vi "ref_forcecontrol_pitchmotor_pid_sensor.vi"() -> ()   [LabVIEW 2014]
uses:
  <vilib>/rvi/FXPMathLib/FxpSinAndCos/XNode/nifxpmath_SinAndCos.xnode
  <vilib>/eio/EIONode/EIONode.xnode
  <vilib>/rvi/FXPMathLib/FxpMul/XNode/nifxpmath_Multiplier.xnode
  <vilib>/rvi/FXPMathLib/FxpSinAndCos/simVIs/DllFxpSinAndCosTemp_sub.vi
  <vilib>/rvi/FXPMathLib/FxpSinAndCos/subVIs/nifxpmath_SinAndCos_SimConfig.ctl
  <vilib>/rvi/eio/common/nirviEmuTemplateMethod_errors.vi
  <vilib>/rvi/FXPMathLib/sim/FxpSim.dll
  <vilib>/rvi/DataTransferAndStorage/Container/XNode/niFpgaContainer.xnode
  <vilib>/rvi/FXPMathLib/FxpSub/XNode/nifxpmath_Sub.xnode
  <vilib>/rvi/FXPMathLib/FxpAdd/XNode/nifxpmath_Add.xnode
  <vilib>/rvi/Analysis/measure/butterworth/XNode/niFpgaButterworthFilter.xnode
  <vilib>/eio/EIOPropertyNode/EIOPropertyNode.xnode
  <vilib>/rvi/eio/common/nirviEmuTemplatePropertyGet_errors.vi
  <vilib>/rvi/eio/common/nirviEmuTemplatePropertyGet_noerrors.vi
  <vilib>/rvi/eio/common/nirviEmuTemplatePropertySet_errors.vi
  <vilib>/rvi/eio/common/nirviEmuTemplatePropertySet_noerrors.vi
  <vilib>/rvi/interface/RandomDataEmulation/nirviRandomDataFpgaReadWriteTemplate.vi
  <vilib>/LabVIEW Targets/FPGA/cRIO/shared/nicrio_ModuleControls/nicrio_cRIO-9237_DataRatesRing.ctl
  <vilib>/LabVIEW Targets/FPGA/cRIO/shared/nicrio_ModuleControls/nicrio_cRIO-9237_ExcitationVoltageRing.ctl
panel:
  in  "Unstrained Measurements_p":fxp<+/-,22,1>
  in  "LRCF_p":fxp<+,22,1>
  in  "Unstrained Measurements_y":fxp<+/-,22,1>
  in  "LRCF_y":fxp<+,22,1>
  in  "Fey_reset":bool
  out "Gauge_Fey":fxp<+/-,24,-4>
  in  "Gauge_stop":bool
  in  "Fep_reset":bool
  out "Gauge_Fep":fxp<+/-,24,-4>
  in  "Excitation Voltage":T1 items=["2.5 Volts", "3.3 Volts", "5.0 Volts", "10.0 Volts", "External Excitation"]
  in  "Data Rate":T2=1 items=["50.000 kS/s (NI 9237)"=1, "25.000 kS/s (NI 9237)"=2, "16.667 kS/s (NI 9237)"=3, "12.500 kS/s (NI 9237)"=4, "10.000 kS/s (NI 9237)"=5, "8.333 kS/s (NI 9237)"=6, "7.143 kS/s (NI 9237)"=7, "6.250 kS/s (NI 9237)"=8, "5.556 kS/s (NI 9237)"=9, "5.000 kS/s (NI 9237)"=10, "4.545 kS/s (NI 9237)"=11, "4.167 kS/s (NI 9237)"=12, "3.846 kS/s (NI 9237)"=13, "3.571 kS/s (NI 9237)"=14, "3.333 kS/s (NI 9237)"=15, "3.125 kS/s (NI 9237)"=16, "2.941 kS/s (NI 9237)"=17, "2.778 kS/s (NI 9237)"=18, "2.632 kS/s (NI 9237)"=19, "2.500 kS/s (NI 9237)"=20, "2.381 kS/s (NI 9237)"=21, "2.273 kS/s (NI 9237)"=22, "2.174 kS/s (NI 9237)"=23, "2.083 kS/s (NI 9237)"=24, "2.000 kS/s (NI 9237)"=25, "1.923 kS/s (NI 9237)"=26, "1.852 kS/s (NI 9237)"=27, "1.786 kS/s (NI 9237)"=28, "1.724 kS/s (NI 9237)"=29, "1.667 kS/s (NI 9237)"=30, "1.613 kS/s (NI 9237)"=31]
  in  "Step_fp_start":bool
  in  "Count(mSec)":u32
  in  "Fpr_step":fxp<+/-,20,10>
  in  "Fpr_numofstep":i32
  in  "Fpr_ini":fxp<+/-,20,10>
  in  "coe_ini":bool
  in  "D_comp/tune_p":bool
  in  "kp t":fxp<+,15,8>
  in  "kp c":fxp<+,15,8>
  in  "Kpp gain":fxp<+,10,4>=0.40625
  in  "Kpp slope gain":fxp<+,20,1>=0.40625
  in  "Kdp 2":fxp<+,26,2>
  in  "Kip 2":fxp<+,27,10>
  in  "I_comp/tune_p":bool
  out "Kpp":fxp<+,12,6>
  out "Kdp":fxp<+,26,2> format="%.25g"
  out "Kip":fxp<+,27,10> format="%.21g"
  in  "tolerance_p":fxp<+,12,2>=1.0
  out "fpr":fxp<+/-,20,10>
  in  "viscous_cons_p":fxp<+/-,20,10>
  in  "fcp":fxp<+/-,15,6>
  in  "fvp":fxp<+,20,12>
  in  "fv_coeff. p":fxp<+,13,1>
  in  "Dp_d_tol":fxp<+,20,12>
  in  "fstp":fxp<+/-,15,6>
  out "Friction comp_p":fxp<+/-,20,10>
  out "Fp_PID":fxp<+/-,20,10>
  out "fp_tilde":fxp<+/-,21,11>
  out "fpt_d":fxp<+/-,25,15>
  out "xp_d":fxp<+/-,25,15>
  out "fpt_i":fxp<+/-,25,11>
  out "Dp_d":fxp<+/-,25,15>
  out "vd_p_F":fxp<+/-,20,5>
  out "vq_p_F":fxp<+/-,20,5> format="%.57g"
  in  "Stop motor_p":bool
  out "va_p":fxp<+/-,20,5> format="%.21g"
  out "vb_p":fxp<+/-,20,5> format="%.21g"
  out "omega_p":fxp<+/-,20,9>
  in  "Encoder Reset_p":bool
  out "Encoder Position_p":i32
  out "rad(NrTheta)_p":fxp<+/-,33,18> format="%.21g"
  out "Dp(mm)":fxp<+/-,22,7>
  out "x_p":fxp<+/-,30,6> format="%.40g"
  in  "Linear Sensor Reset":bool
  in  "kp":fxp<+,15,8>
  out "fp":fxp<+/-,20,10>
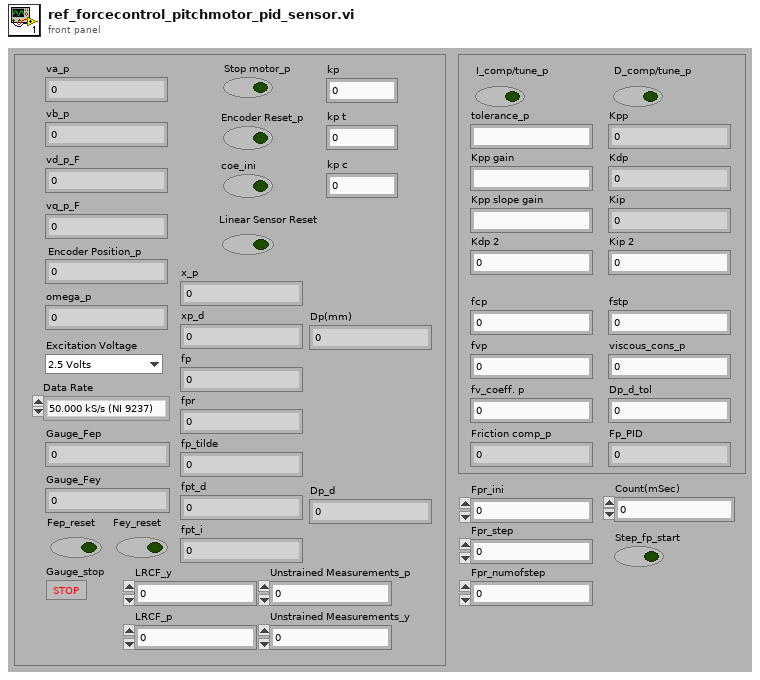
[diagram p1: front panel]
types:
  T1 = typedef "nicrio_cRIO-9237_ExcitationVoltageRing.ctl" = u8
  T2 = typedef "nicrio_cRIO-9237_DataRatesRing.ctl" = u8
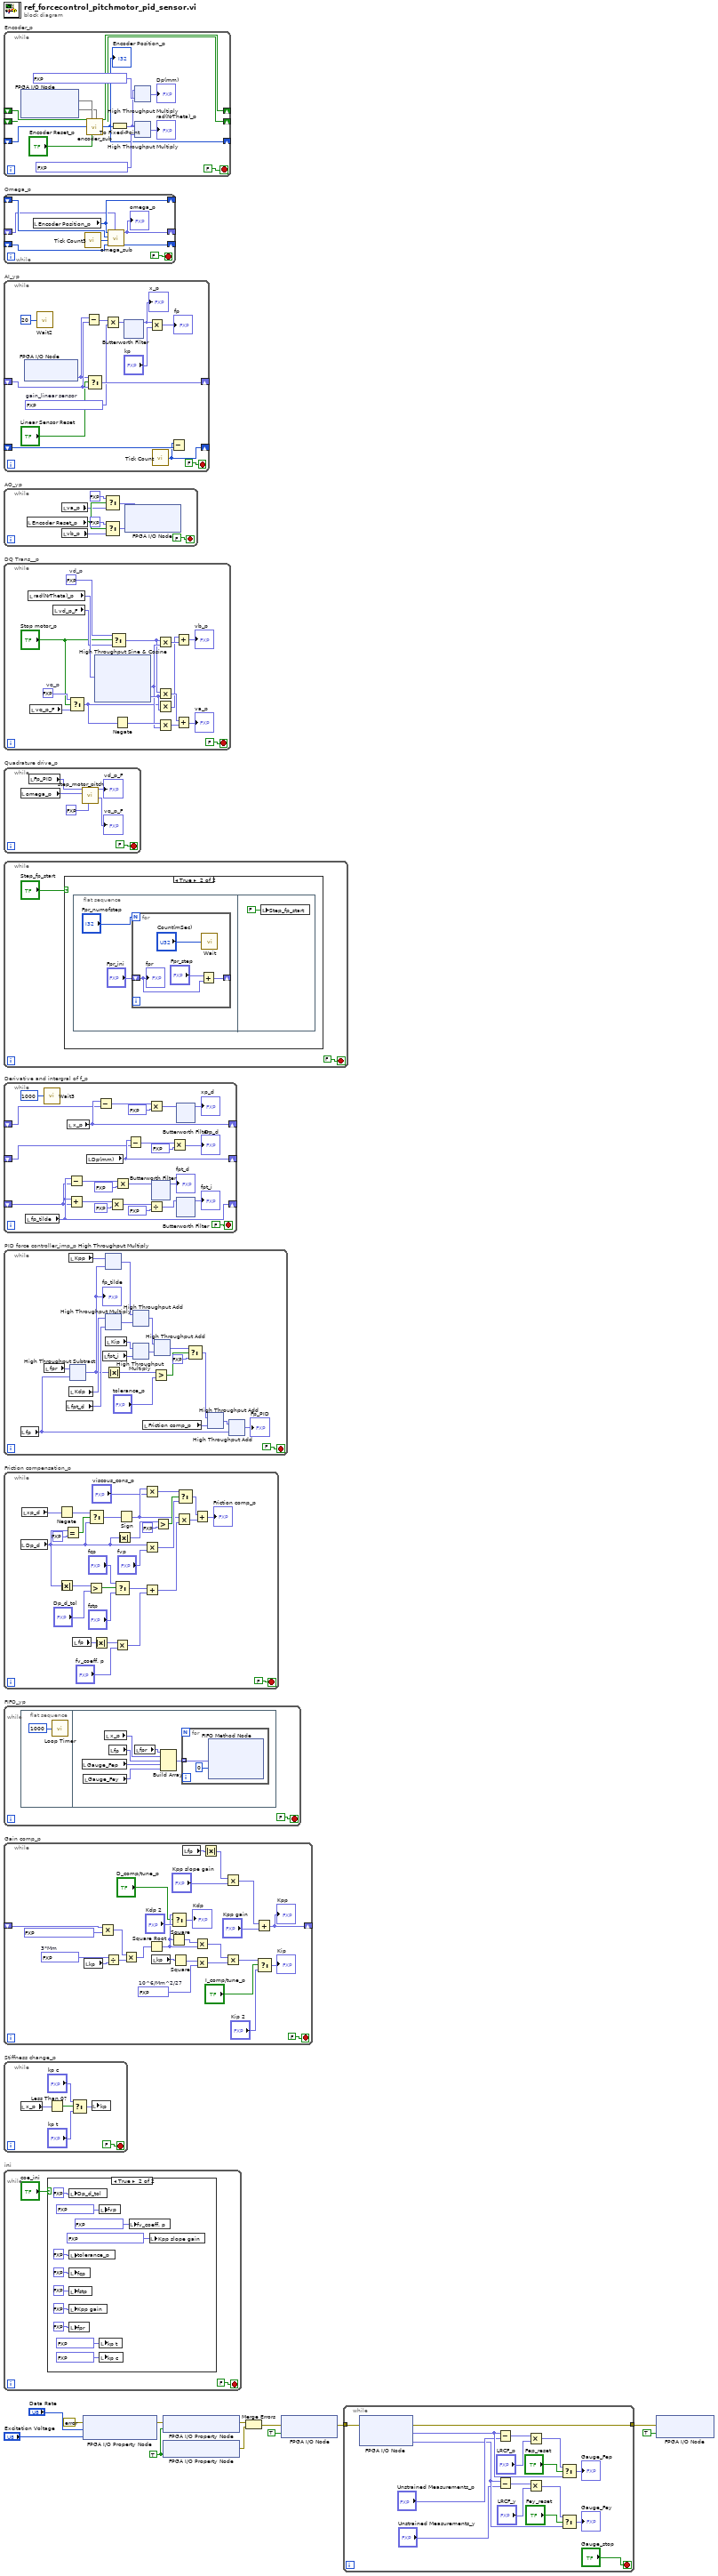
[diagram p0: block diagram]
diagram:
  w6 = TRUE ("Half-Bridge Enable")
  n1 = while "Encoder_p" {
    shift-right: [w26] -> _
    shift-left: _ -> [w24]
    shift-right: [w25] -> _
    shift-left: _ -> [w23]
    shift-right: [w13] -> _
    shift-left: _ -> [w19]
    stop <- FALSE stop-if-true
    n2 = xnode "FPGA I/O Node"() -> ("Mod3/DIO0"=w22, "Mod3/DIO1"=w21)  [unwired: 2 in, 2 out]
    n3 = call "encoder_sub.vi"("A_pre"=w24, "B_pre"=w23, "Encoder Position_pre"=w19, "A input"=w22, "Encoder Position Reset"="Encoder Reset_p", "B input"=w21) -> ("A"=w26:bool, "B"=w25:bool, "Encoder Position (Counts)"=w13:i32)  [unwired: 19 in]
    "Encoder Position_p" <- w13
    n4 = To Fixed-Point(number=w13) -> (fixed-point=w16:fxp<+/-,18,18>)  [unwired: 1 in]
    n5 = xnode ("High Throughput Multiply")("x"=w16, "y"=fxp<+/-,15,-9> -0.0006049871444702148) -> ("x*y"=→"Dp(mm)":fxp<+/-,21,6>)
    n6 = xnode ("High Throughput Multiply")("x"=w16, "y"=fxp<+,24,0> 0.02499997615814209) -> ("x*y"=→"rad(NrTheta)_p":fxp<+/-,33,18>)
  }
  n7 = while "Omega_p" {
    shift-right: [w35] -> _
    shift-left: _ -> [w34]
    shift-right: [w33] -> _
    shift-left: _ -> [w32]
    shift-right: [w30] -> _
    shift-left: _ -> [w31]
    stop <- FALSE stop-if-true
    n8 = local read "Encoder Position_p"() -> (w35:i32)
    n9 = call "Tick Count3"() -> ("Tick Count(Ticks)"=w28:u32)
    n10 = call "omega_sub.vi"("omega_pre"=w31, "ticks_m_pre"=w32, "ticks"=w28, "count_pre"=w34, "count"=w35) -> ("ticks_m"=w33:u32, "omega"=w30:fxp<+/-,20,9>)  [unwired: 4 in, 1 out]
    "omega_p" <- w30
  }
  n11 = while "AI_yp" {
    shift-right: [w48] -> _
    shift-left: _ -> [w49]
    shift-right: [w45] -> _
    shift-left: _ -> [w46]
    stop <- FALSE stop-if-true
    w36 = fxp<+,25,5> 1.4694995880126953  # gain_linear sensor
    n12 = xnode "FPGA I/O Node"() -> ("Mod1/AI0"=w42:fxp<+/-,20,5>)  [unwired: 2 in, 2 out]
    n13 = call "Wait2"("Count(uSec)"=u8 20) -> ()  [unwired: 1 out]
    n14 = Subtract(x=w42, y=w46) -> (x-y=w40:fxp<+/-,21,6>)
    n15 = Select(t=w42, s="Linear Sensor Reset", f=w46) -> (s? t:f=w45:fxp<+/-,20,5>)
    n16 = Multiply(x=w40, y=w36) -> (x*y=w38:fxp<+/-,30,6>)
    n17 = xnode "Butterworth Filter"("input data"=w38) -> ("output data"=w37:fxp<+/-,30,6>)  [unwired: 2 in]
    "x_p" <- w37
    n18 = Multiply(x=w37, y="kp") -> (x*y=→"fp":fxp<+/-,20,10>)
    n19 = call "Tick Count"() -> ("Tick Count(uSec)"=w48:u8)
    n20 = Subtract(x=w48, y=w49) -> ()  [unwired: 1 out]
  }
  n21 = while "AO_yp" {
    stop <- FALSE stop-if-true
    n22 = local read "Encoder Reset_p"() -> (w64:bool)
    n23 = local read "va_p"() -> (w63:fxp<+/-,20,5>)
    n24 = local read "vb_p"() -> (w62:fxp<+/-,20,5>)
    n25 = Select(t=fxp<+/-,20,5> 5.0 ("Mod2/AO4"), s=w64, f=w63) -> (s? t:f=w59:fxp<+/-,20,5>)
    n26 = Select(t=fxp<+/-,20,5> 0.0 ("Mod2/AO4"), s=w64, f=w62) -> (s? t:f=w58:fxp<+/-,20,5>)
    n27 = xnode "FPGA I/O Node"("Mod2/AO0"=w59, "Mod2/AO1"=w58) -> ()  [unwired: 2 in, 2 out]
  }
  n28 = while "DQ Trans__p" {
    stop <- FALSE stop-if-true
    w73 = fxp<+/-,20,5> 0.0  # vq_p
    w71 = fxp<+/-,20,5> 0.0  # vd_p
    n29 = local read "rad(NrTheta)_p"() -> (w82:fxp<+/-,33,18>)
    n30 = local read "vq_p_F"() -> (w69:fxp<+/-,20,5>)
    n31 = local read "vd_p_F"() -> (w70:fxp<+/-,20,5>)
    n32 = Select(t=w73, s="Stop motor_p", f=w69) -> (s? t:f=w74:fxp<+/-,20,5>)
    n33 = xnode "High Throughput Sine & Cosine"("x (pi)"=w82) -> ("sin(x)"=w75:fxp<+/-,17,2>, "cos(x)"=w76:fxp<+/-,17,2>)
    n34 = Select(t=w71, s="Stop motor_p", f=w70) -> (s? t:f=w72:fxp<+/-,20,5>)
    n35 = Negate(x=w74) -> (-x=w81:fxp<+/-,21,6>)
    n36 = Multiply(x=w72, y=w75) -> (x*y=w78:fxp<+/-,20,5>)
    n37 = Multiply(x=w72, y=w76) -> (x*y=w80:fxp<+/-,20,5>)
    n38 = Multiply(x=w74, y=w76) -> (x*y=w77:fxp<+/-,20,5>)
    n39 = Multiply(x=w81, y=w75) -> (x*y=w79:fxp<+/-,20,5>)
    n40 = Add(x=w77, y=w78) -> (x+y=→"vb_p":fxp<+/-,20,5>)
    n41 = Add(x=w80, y=w79) -> (x+y=→"va_p":fxp<+/-,20,5>)
  }
  n42 = while "Quadrature drive_p" {
    stop <- FALSE stop-if-true
    n43 = local read "omega_p"() -> (w116:fxp<+/-,20,9>)
    n44 = local read "Fp_PID"() -> (w118:fxp<+/-,20,10>)
    n45 = call "step_motor_pitch.vi"("F_Threshold"=fxp<+,12,12> 10.0, "omega_p"=w116, "F"=w118) -> ("vq_F"=→"vq_p_F":fxp<+/-,20,5>, "vd_F"=→"vd_p_F":fxp<+/-,20,5>)  [unwired: 7 in]
  }
  n46 = while {
    stop <- FALSE stop-if-true
    n47 = case shown="True" "Step_fp_start" {
      frame False {
      }
      frame True {
        n48 = flat-sequence {
          frame #0 {
            n49 = for {
              N: "Fpr_numofstep" -> [_]
              shift-right: [w125] -> _
              shift-left: "Fpr_ini" -> [w126]
              n50 = Add(x="Fpr_step", y=w126) -> (x+y=w125:fxp<+/-,21,11>)
              n51 = call "Wait"("Count(mSec)"="Count(mSec)") -> ()  [unwired: 1 out]
              "fpr" <- w126
            }
          }
          frame #1 {
            n52 = local write "Step_fp_start"(FALSE ("Step_fp_start")) -> ()
          }
        }
      }
    }
  }
  n53 = while "Derivative and intergral of f_p" {
    shift-right: [w141] -> _
    shift-left: _ -> [w140]
    shift-right: [w144] -> _
    shift-left: _ -> [w143]
    shift-right: [w131] -> _
    shift-left: _ -> [w130]
    stop <- FALSE stop-if-true
    n54 = local read "fp_tilde"() -> (w141:fxp<+/-,21,11>)
    n55 = call "Wait3"("Count(uSec)"=u32 1000 ("Count(mSec)")) -> ()  [unwired: 1 out]
    n56 = local read "x_p"() -> (w144:fxp<+/-,30,6>)
    n57 = Subtract(x=w141, y=w140) -> (x-y=w150:fxp<+/-,22,12>)
    n58 = Add(x=w141, y=w140) -> (x+y=w139:fxp<+/-,22,12>)
    n59 = local read "Dp(mm)"() -> (w131:fxp<+/-,22,7>)
    n60 = Subtract(x=w144, y=w143) -> (x-y=w146:fxp<+/-,31,7>)
    n61 = Multiply(x=w139, y=fxp<+/-,22,12> 0.5) -> (x*y=w137:fxp<+/-,25,15>)
    n62 = Multiply(x=w150, y=fxp<+,10,10> 1000.0) -> (x*y=w149:fxp<+/-,25,15>)
    n63 = Subtract(x=w131, y=w130) -> (x-y=w133:fxp<+/-,23,8>)
    n64 = Multiply(x=w146, y=fxp<+,10,10> 1000.0) -> (x*y=w145:fxp<+/-,25,15>)
    n65 = Divide(x=w137, y=fxp<+/-,25,15> 1000.0) -> (x/y=w135:fxp<+/-,25,11>)
    n66 = xnode "Butterworth Filter"("input data"=w149) -> ("output data"=→"fpt_d":fxp<+/-,25,15>)  [unwired: 2 in]
    n67 = Multiply(x=w133, y=fxp<+,10,10> 1000.0) -> (x*y=→"Dp_d":fxp<+/-,25,15>)
    n68 = xnode "Butterworth Filter"("input data"=w145) -> ("output data"=→"xp_d":fxp<+/-,25,15>)  [unwired: 2 in]
    n69 = xnode "Butterworth Filter"("input data"=w135) -> ("output data"=→"fpt_i":fxp<+/-,25,11>)  [unwired: 2 in]
  }
  n70 = while "PID force controller_imp_p" {
    stop <- FALSE stop-if-true
    n71 = local read "fp"() -> (w190:fxp<+/-,20,10>)
    n72 = local read "fpr"() -> (w179:fxp<+/-,20,10>)
    n73 = local read "fpt_d"() -> (w191:fxp<+/-,25,15>)
    n74 = local read "Kpp"() -> (w193:fxp<+,12,6>)
    n75 = local read "Kdp"() -> (w192:fxp<+,26,2>)
    n76 = xnode "High Throughput Subtract"("x"=w179, "y"=w190) -> ("x-y"=w184:fxp<+/-,21,11>)
    "fp_tilde" <- w184
    n77 = local read "fpt_i"() -> (w188:fxp<+/-,25,11>)
    n78 = xnode ("High Throughput Multiply")("x"=w193, "y"=w184) -> ("x*y"=w194:fxp<+/-,33,17>)
    n79 = xnode ("High Throughput Multiply")("x"=w192, "y"=w191) -> ("x*y"=w183:fxp<+/-,31,21>)
    n80 = local read "Kip"() -> (w187:fxp<+,27,10>)
    n81 = Absolute Value(x=w184) -> (abs(x)=w197:fxp<+,21,11>)
    n82 = xnode ("High Throughput Add")("x"=w194, "y"=w183) -> ("x+y"=w189:fxp<+/-,20,10>)
    n83 = xnode ("High Throughput Multiply")("x"=w187, "y"=w188) -> ("x*y"=w186:fxp<+/-,31,14>)
    n84 = local read "Friction comp_p"() -> (w180:fxp<+/-,20,10>)
    n85 = Greater?(x=w197, y="tolerance_p") -> (0:w196:bool)
    n86 = xnode ("High Throughput Add")("x"=w189, "y"=w186) -> ("x+y"=w185:fxp<+/-,20,10>)
    n87 = Select(t=w185, s=w196, f=fxp<+/-,20,10> 0.0) -> (s? t:f=w182:fxp<+/-,20,10>)
    n88 = xnode ("High Throughput Add")("x"=w182, "y"=w180) -> ("x+y"=w181:fxp<+/-,20,10>)
    n89 = xnode ("High Throughput Add")("x"=w181, "y"=w190) -> ("x+y"=→"Fp_PID":fxp<+/-,20,10>)
  }
  n90 = while "Friction compensation_p" {
    stop <- FALSE stop-if-true
    n91 = local read "Dp_d"() -> (w206:fxp<+/-,25,15>)
    n92 = local read "xp_d"() -> (w201:fxp<+/-,25,15>)
    n93 = Negate(x=w201) -> (-x=w200:fxp<+/-,26,16>)
    n94 = Absolute Value(x=w206) -> (abs(x)=w219:fxp<+,25,15>)
    n95 = Equal?(x=w206, y=fxp<+/-,25,15> 0.0) -> (x = y?=w207:bool)
    n96 = local read "fp"() -> (w224:fxp<+/-,20,10>)
    n97 = Greater?(x=w219, y="Dp_d_tol") -> (0:w218:bool)
    n98 = Select(t=w200, s=w207, f=w206) -> (s? t:f=w205:fxp<+/-,26,16>)
    n99 = Absolute Value(x=w224) -> (abs(x)=w225:fxp<+,20,10>)
    n100 = Select(t="fcp", s=w218, f="fstp") -> (s? t:f=w216:fxp<+/-,15,6>)
    n101 = Multiply(x=w225, y="fv_coeff. p") -> (x*y=w223:fxp<+/-,20,10>)
    n102 = Absolute Value(x=w206) -> (abs(x)=w213:fxp<+,25,15>)
    n103 = Sign(1:w205) -> (0:w204:fxp<+/-,2,2>)
    n104 = Multiply(x=w204, y="viscous_cons_p") -> (x*y=w209:fxp<+/-,20,10>)
    n105 = Multiply(x=w206, y="fvp") -> (x*y=w211:fxp<+/-,20,10>)
    n106 = Add(x=w216, y=w223) -> (x+y=w222:fxp<+/-,20,10>)
    n107 = Greater?(x=w213, y=fxp<+/-,25,15> 25.0) -> (0:w212:bool)
    n108 = Multiply(x=w204, y=w222) -> (x*y=w221:fxp<+/-,20,10>)
    n109 = Select(t=w209, s=w212, f=w211) -> (s? t:f=w210:fxp<+/-,20,10>)
    n110 = Add(x=w210, y=w221) -> (x+y=→"Friction comp_p":fxp<+/-,20,10>)
  }
  n111 = while "FIFO_yp" {
    stop <- FALSE stop-if-true
    n112 = flat-sequence {
      frame #0 {
        n113 = call "Loop Timer"("Count(uSec)"=u32 1000 ("Loop Period (usec)")) -> ()  [unwired: 1 out]
      }
      frame #1 {
        n114 = local read "Gauge_Fep"() -> (w233:fxp<+/-,24,-4>)
        n115 = local read "Gauge_Fey"() -> (w232:fxp<+/-,24,-4>)
        n116 = local read "x_p"() -> (w235:fxp<+/-,30,6>)
        n117 = local read "fp"() -> (w234:fxp<+/-,20,10>)
        n118 = local read "fpr"() -> (w236:fxp<+/-,20,10>)
        n119 = Build Array(w236, w235, w234, w233, w232) -> (w231:fxp<+/-,38,10>[])
        n120 = for {
          tunnel: w231 -> [w237] mode=indexing
          n121 = xnode ("FIFO Method Node")("Element"=w237, "Timeout"=0) -> ()  [unwired: 1 in, 2 out]
        }
      }
    }
  }
  n122 = while "Gain comp_p" {
    shift-right: [w243] -> _
    shift-left: _ -> [w262]
    stop <- FALSE stop-if-true
    w250 = fxp<+,14,7> 111.8125  # 10^6/Mm^2/27
    w265 = fxp<+,14,7> 54.6015625  # 3*Mm
    n123 = local read "kp"() -> (w264:fxp<+,15,8>)
    n124 = Multiply(x=w262, y=fxp<+,12,-6> 0.00099945068359375) -> (x*y=w261:fxp<+,24,0>)
    n125 = Divide(x=w265, y=w264) -> (x/y=w260:fxp<+,23,7>)
    n126 = Multiply(x=w261, y=w260) -> (x*y=w259:fxp<+,32,0>)
    n127 = Square Root(x=w259) -> (sqrt(x)=w246:fxp<+,26,2>)
    n128 = local read "kp"() -> (w251:fxp<+,15,8>)
    n129 = Square(x=w246) -> (x^2=w253:fxp<+,27,3>)
    n130 = Select(t=w246, s="D_comp/tune_p", f="Kdp 2") -> (s? t:f=→"Kdp":fxp<+,26,2>)
    n131 = Square(x=w251) -> (x^2=w249:fxp<+,30,16>)
    n132 = local read "fp"() -> (w256:fxp<+/-,20,10>)
    n133 = Multiply(x=w253, y=w246) -> (x*y=w252:fxp<+,27,3>)
    n134 = Multiply(x=w249, y=w250) -> (x*y=w248:fxp<+,44,20>)
    n135 = Absolute Value(x=w256) -> (abs(x)=w257:fxp<+,20,10>)
    n136 = Multiply(x=w257, y="Kpp slope gain") -> (x*y=w255:fxp<+,12,4>)
    n137 = Multiply(x=w252, y=w248) -> (x*y=w245:fxp<+,27,10>)
    n138 = Add(x=w255, y="Kpp gain") -> (x+y=w243:fxp<+,12,6>)
    "Kpp" <- w243
    n139 = Select(t=w245, s="I_comp/tune_p", f="Kip 2") -> (s? t:f=→"Kip":fxp<+,27,10>)
  }
  n140 = while "Stiffness change_p" {
    stop <- FALSE stop-if-true
    n141 = local read "x_p"() -> (w267:fxp<+/-,30,6>)
    n142 = Less Than 0?(x=w267) -> (x < 0?=w268:bool)
    n143 = Select(t="kp c", s=w268, f="kp t") -> (s? t:f=w269:fxp<+,15,8>)
    n144 = local write "kp"(w269) -> ()
  }
  n145 = while "ini" {
    stop <- FALSE stop-if-true
    n146 = case shown="True" "coe_ini" {
      frame False {
      }
      frame True {
        n147 = local write "Dp_d_tol"(fxp<+,20,12> 3.0 ("Dp_d_tol")) -> ()
        n148 = local write "tolerance_p"(fxp<+,12,2> 1.0 ("tolerance_p")) -> ()
        n149 = local write "fcp"(fxp<+/-,15,6> 6.0 ("fcp")) -> ()
        n150 = local write "fstp"(fxp<+/-,15,6> 8.0 ("fstp")) -> ()
        n151 = local write "Kpp gain"(fxp<+,10,4> 3.0 ("Kpp gain")) -> ()
        n152 = local write "fpr"(fxp<+/-,20,10> 0.0 ("fpr")) -> ()
        n153 = local write "fvp"(fxp<+,20,12> 0.19921875 ("fvp")) -> ()
        n154 = local write "kp t"(fxp<+,15,8> 31.8046875 ("kp t")) -> ()
        n155 = local write "kp c"(fxp<+,15,8> 36.2421875 ("kp c")) -> ()
        n156 = local write "fv_coeff. p"(fxp<+,13,1> 0.14990234375 ("fv_coeff. p")) -> ()
        n157 = local write "Kpp slope gain"(fxp<+,20,1> 0.14999961853027344 ("Kpp slope gain")) -> ()
      }
    }
  }
  n158 = xnode "FPGA I/O Property Node"("error in"=errorcluster {"status"=FALSE, "code"=0, "source"=""}, "Data Rate"="Data Rate", "Excitation Voltage"="Excitation Voltage") -> ("error out"=w8:errorcluster)  [unwired: 1 in, 1 out]
  n159 = xnode "FPGA I/O Property Node"("error in"=w8, "Half-Bridge Enable"=w6) -> ("error out"=w5:errorcluster)  [unwired: 1 in, 1 out]
  n160 = xnode "FPGA I/O Property Node"("Half-Bridge Enable"=w6) -> ("error out"=w4:errorcluster)  [unwired: 2 in, 1 out]
  n161 = Merge Errors(w5, w4) -> (w3:errorcluster)
  n162 = xnode "FPGA I/O Node"("error in"=w3, "Mod6/Start"=TRUE ("Mod4/Start")) -> ("error out"=w2:errorcluster)  [unwired: 1 in, 1 out]
  n163 = while {
    tunnel: w2 -> [w301]
    tunnel: [w302] -> w1
    stop <- "Gauge_stop" stop-if-true
    n164 = xnode "FPGA I/O Node"("error in"=w301) -> ("error out"=w302:errorcluster, "Mod6/AI0"=w300:fxp<+/-,24,-4>, "Mod6/AI1"=w295:fxp<+/-,24,-4>)  [unwired: 2 in, 2 out]
    n165 = Subtract(x=w300, y="Unstrained Measurements_p") -> (x-y=w298:fxp<+/-,30,2>)
    n166 = Subtract(x=w295, y="Unstrained Measurements_y") -> (x-y=w293:fxp<+/-,30,2>)
    n167 = Multiply(x=w298, y="LRCF_p") -> (x*y=w296:fxp<+/-,24,-4>)
    n168 = Multiply(x=w293, y="LRCF_y") -> (x*y=w291:fxp<+/-,24,-4>)
    n169 = Select(t=w296, s="Fep_reset", f=w300) -> (s? t:f=→"Gauge_Fep":fxp<+/-,24,-4>)
    n170 = Select(t=w291, s="Fey_reset", f=w295) -> (s? t:f=→"Gauge_Fey":fxp<+/-,24,-4>)
  }
  n171 = xnode "FPGA I/O Node"("error in"=w1, "Mod6/Stop"=TRUE ("Mod4/Stop")) -> ()  [unwired: 1 in, 2 out]
